vi "Write Wärmepumpe.Parameter.vi"(8 "error in (no error)":errorcluster, 10 "Wärmepumpe.Parameter":T1, 11 "Wärmepumpe in":refnum<class "Wärmepumpe.lvclass">) -> (0 "error out":errorcluster, 3 "Wärmepumpe out":refnum<class "Wärmepumpe.lvclass">)   [LabVIEW 2016, in "Wärmepumpe.lvclass"]
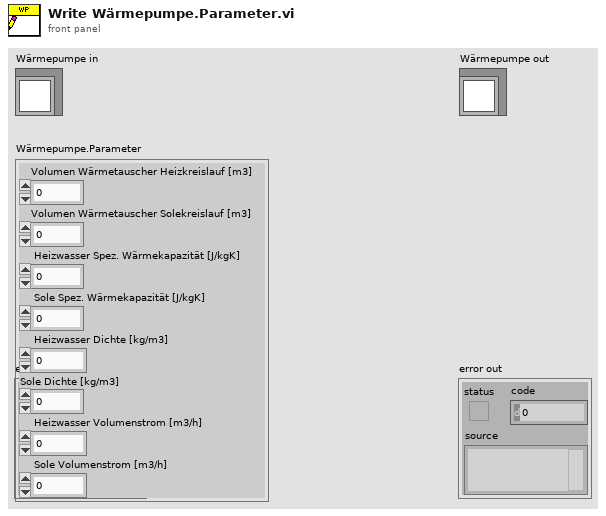
[diagram p1: front panel]
types:
  T1 = cluster{"Volumen Wärmetauscher Heizkreislauf [m3]":dbl, "Volumen Wärmetauscher Solekreislauf [m3]":dbl, " Heizwasser Spez. Wärmekapazität [J/kgK]":dbl, " Sole Spez. Wärmekapazität [J/kgK]":dbl, " Heizwasser Dichte [kg/m3]":dbl, "Sole Dichte [kg/m3] ":dbl, " Heizwasser Volumenstrom [m3/h]":dbl, " Sole Volumenstrom [m3/h]":dbl}
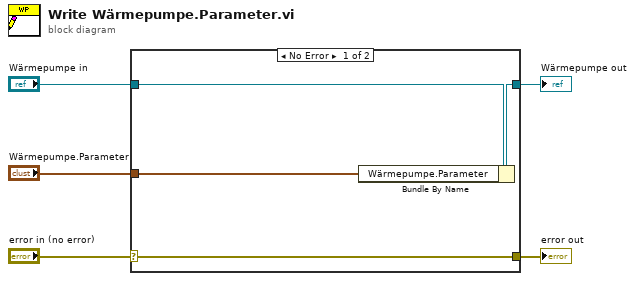
[diagram p0: block diagram]
diagram:
  n1 = case shown="No Error" "error in (no error)" {
    selector: "error in (no error)" -> [w9 w10]
    tunnel: [w9 w10] -> w4
    tunnel: [w7 w11] -> w2
    tunnel: "Wärmepumpe in" -> [w8 w11]
    tunnel: "Wärmepumpe.Parameter" -> [w6 _]
    frame No Error {
      n2 = Bundle By Name(cluster=w8, "Wärmepumpe.Parameter"=w6) -> (w7:refnum<class "Wärmepumpe.lvclass">)
    }
    frame Error {
    }
  }
  "error out" <- w4
  "Wärmepumpe out" <- w2
